vi "GetTimestamp.vi"(4 "Enough Samples to Read":bool, 6 "Elements Remaining":u32, 7 "First Read":bool, 9 "Samples to Read":u32, 10 "Sampling Info":T1, 11 "Time Stamp in":timestamp) -> (3 "Time Stamp out":timestamp)   [LabVIEW 2017, in "cRIOWfmLib.lvlib"]
uses:
  <vilib>/addons/InsightCM/Devices/Shared/Cms/cRIOWfmAcq/cRIOWfmLib.lvlib
  <vilib>/addons/InsightCM/Devices/Shared/Cms/cRIOWfmAcq/subVIs/RIO Wfm Cust Ctrls/rwfm_SamplingInfo.ctl
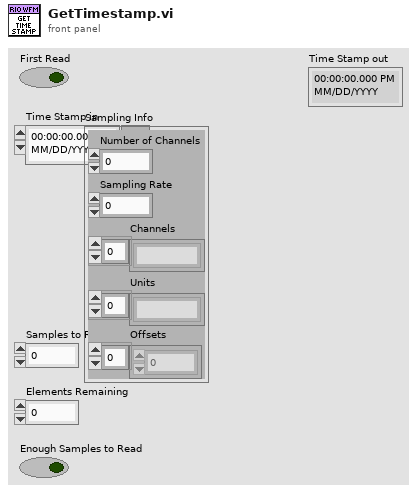
[diagram p1: front panel]
types:
  T1 = typedef "cRIOWfmLib.lvlib/rwfm_SamplingInfo.ctl" = cluster{"Number of Channels":i32, "Sampling Rate":dbl, "Channels":string[], "Units":string[], "Offsets":sgl[]}
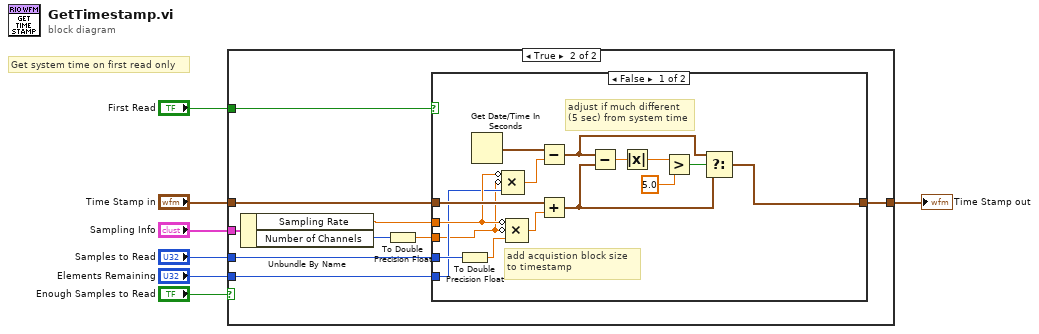
[diagram p0: block diagram]
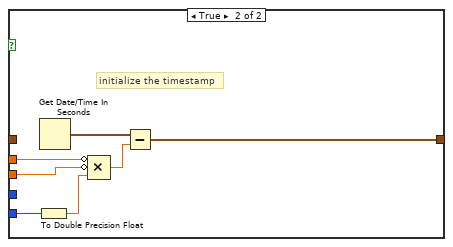
[diagram p3: hidden frame]
diagram:
  # "Get system time on first read only"
  n1 = case shown="True" "Enough Samples to Read" {
    tunnel: "Time Stamp in" -> [w8 w17]
    tunnel: "First Read" -> [_ w16]
    tunnel: "Sampling Info" -> [_ w14]
    tunnel: "Elements Remaining" -> [_ w13]
    tunnel: [w8 w12] -> w5
    tunnel: "Samples to Read" -> [_ w11]
    frame False {
    }
    frame True {
      n2 = Unbundle By Name(w14) -> ("Sampling Rate"=w15:dbl, "Number of Channels"=w10:i32)
      n3 = To Double Precision Float(number=w10) -> (double precision float=w9:dbl)
      n4 = case shown="False" w16 {
        tunnel: w15 -> [w23 w40]
        tunnel: w17 -> [w33 _]
        tunnel: w11 -> [w31 _]
        tunnel: w9 -> [w18 w39]
        tunnel: w13 -> [w22 w36]
        tunnel: [w26 w37] -> w12
        frame False {
          # "adjust if much different (5 sec) from system time"
          # "add acquistion block size\nto timestamp"
          n5 = To Double Precision Float(number=w31) -> (double precision float=w30:dbl)
          n6 = Get Date/Time In Seconds() -> (seconds since 1Jan1904=w24:timestamp)
          n7 = Compound Arithmetic op=MULTIPLY(invert w23, invert w18, w22) -> (w25:dbl)
          n8 = Compound Arithmetic op=MULTIPLY(invert w23, invert w18, w30) -> (w32:dbl)
          n9 = Subtract(x=w24, y=w25) -> (x-y=w21:timestamp)
          n10 = Add(x=w33, y=w32) -> (x+y=w27:timestamp)
          n11 = Subtract(x=w21, y=w27) -> (x-y=w20:dbl)
          n12 = Absolute Value(x=w20) -> (abs(x)=w19:dbl)
          n13 = Greater?(x=w19, y=5.0) -> (0:w28:bool)
          n14 = Select(t=w21, s=w28, f=w27) -> (s? t:f=w26:timestamp)
        }
        frame True {
          # "initialize the timestamp"
          n15 = To Double Precision Float(number=w36) -> (double precision float=w35:dbl)
          n16 = Get Date/Time In Seconds() -> (seconds since 1Jan1904=w34:timestamp)
          n17 = Compound Arithmetic op=MULTIPLY(invert w40, invert w39, w35) -> (w38:dbl)
          n18 = Subtract(x=w34, y=w38) -> (x-y=w37:timestamp)
        }
      }
    }
  }
  "Time Stamp out" <- w5
